vi "spi_control.vi"(0 "connection ID":refnum<k5>, 1 "Device":u16(ring) items=["Attenuation", "Clipping", "Enable channel", "Delay line", "ASIC"], 2 "Read/#write":bool, 3 "Data":i32=72, 4 "Register or channel":i32=72, 5 "error out 3":errorcluster, 6 "Read physical":bool, 7 "Id in":i32, 8 "chip delay":i32) -> (9 "Data to send hex":string, 11 "Data to send dec":u32, 13 "hex integer string":string, 14 "connection ID out":refnum<k5>, 15 "Id out":i32=72, 16 "data out serial":string, 17 "data read value":u32, 19 "error out 2":errorcluster)   [LabVIEW 2009]
panel:
  out "Data out":string
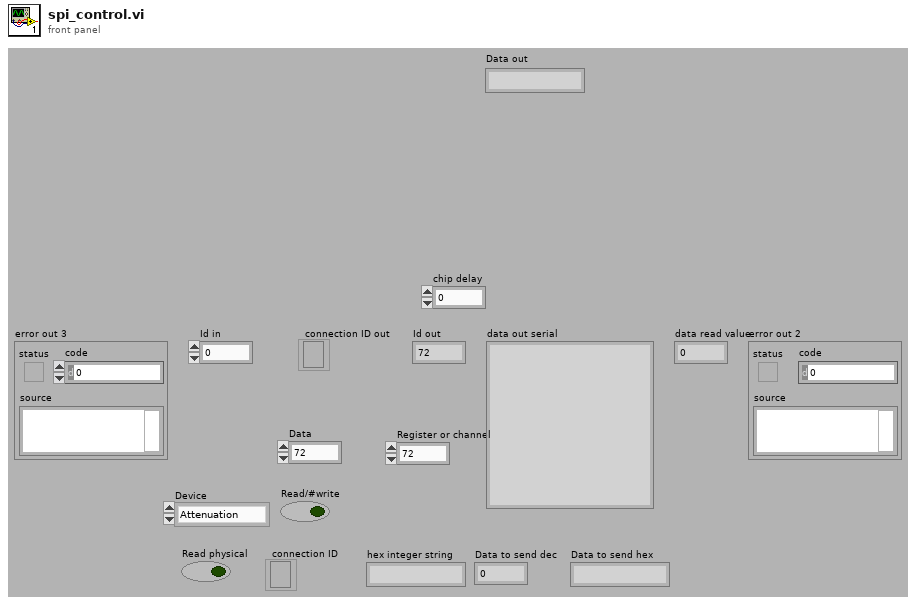
[diagram p1: front panel]
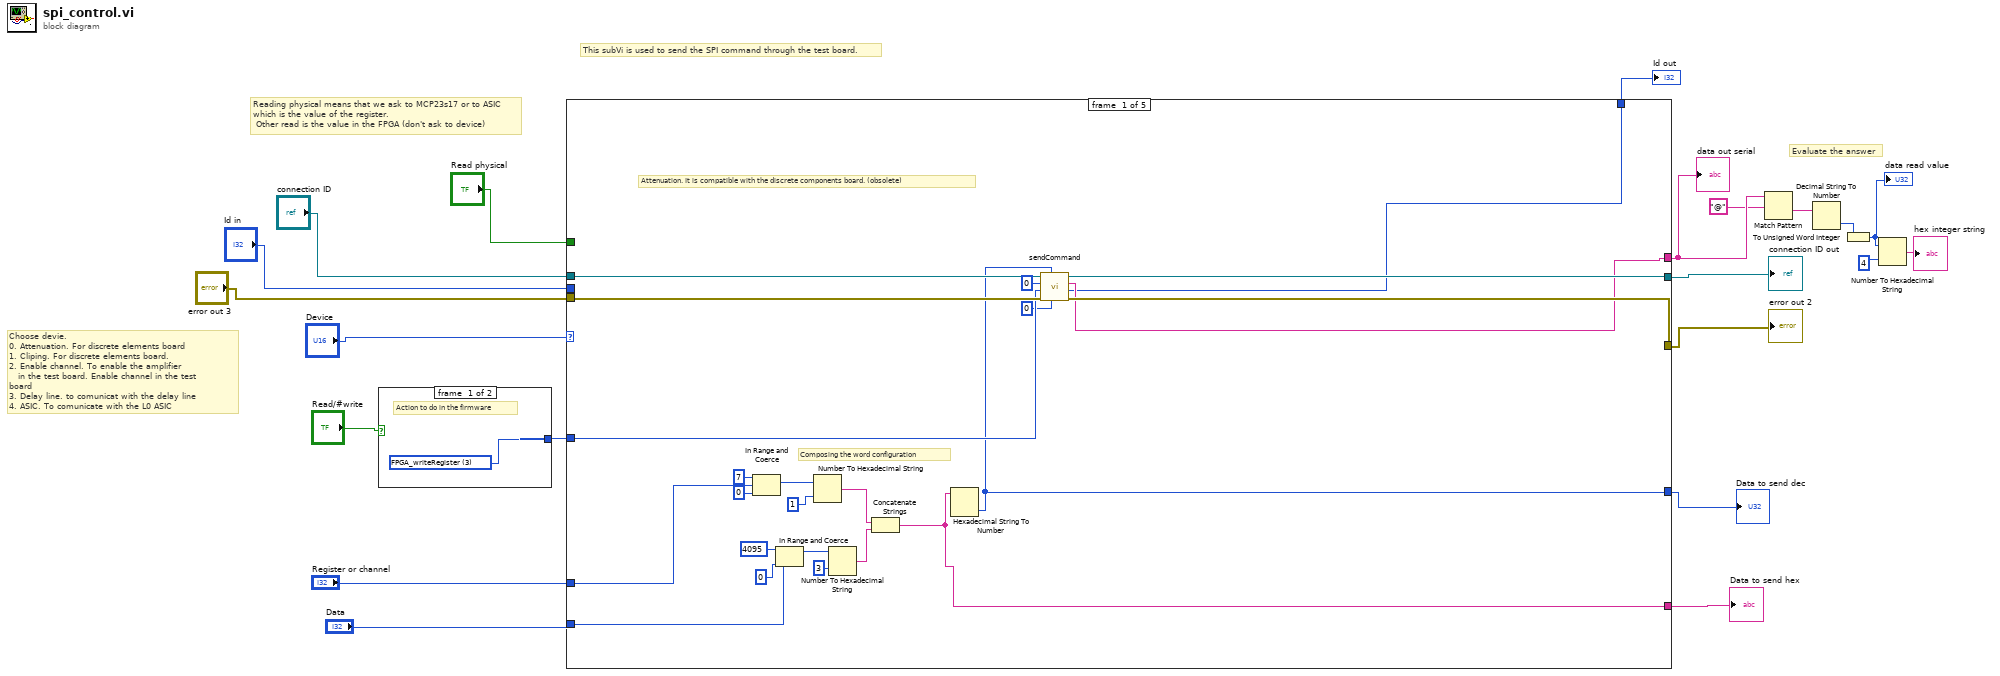
[diagram p0: block diagram]
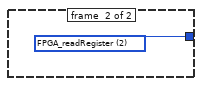
[diagram p2: hidden frame]
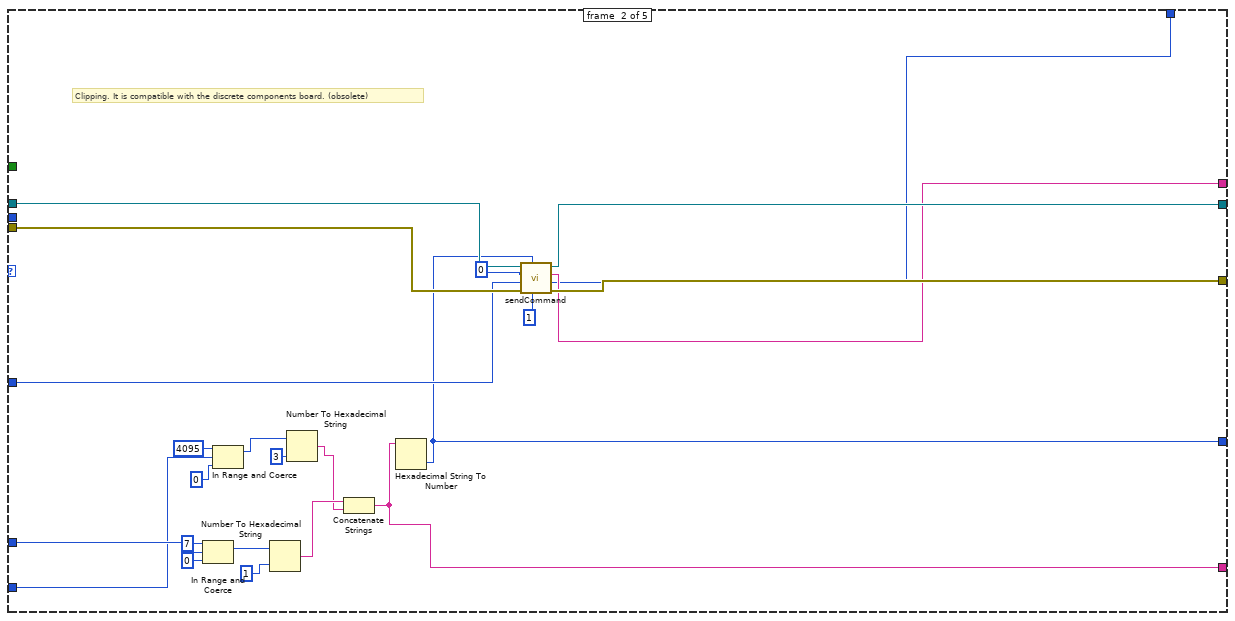
[diagram p3: hidden frame]
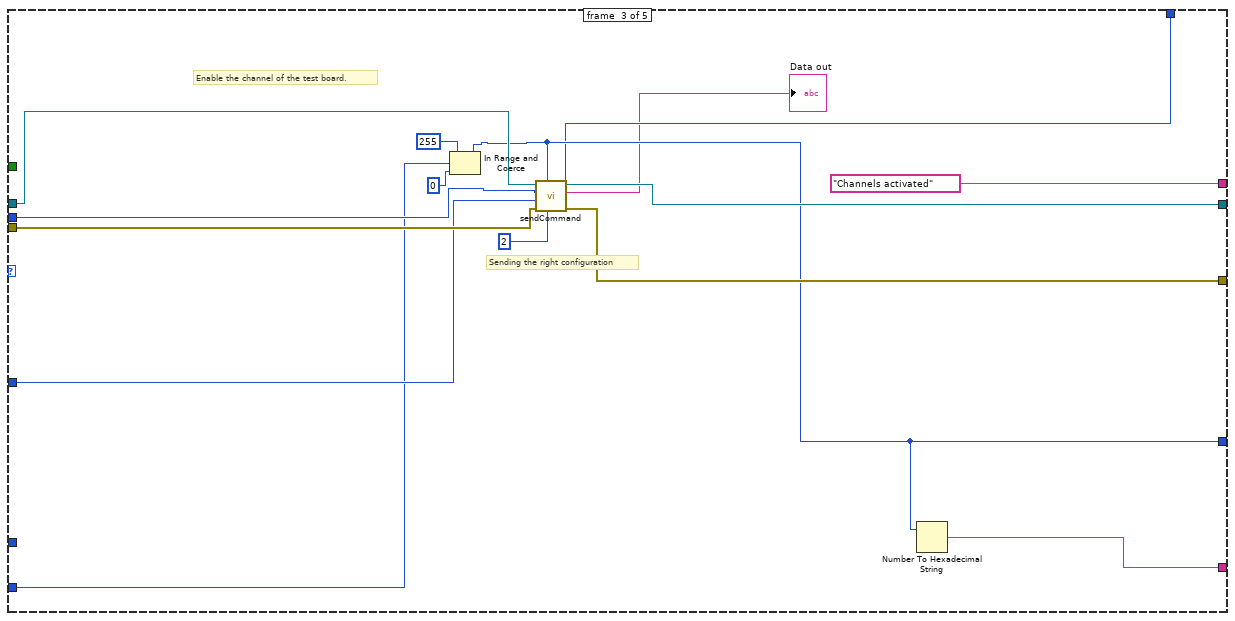
[diagram p4: hidden frame]
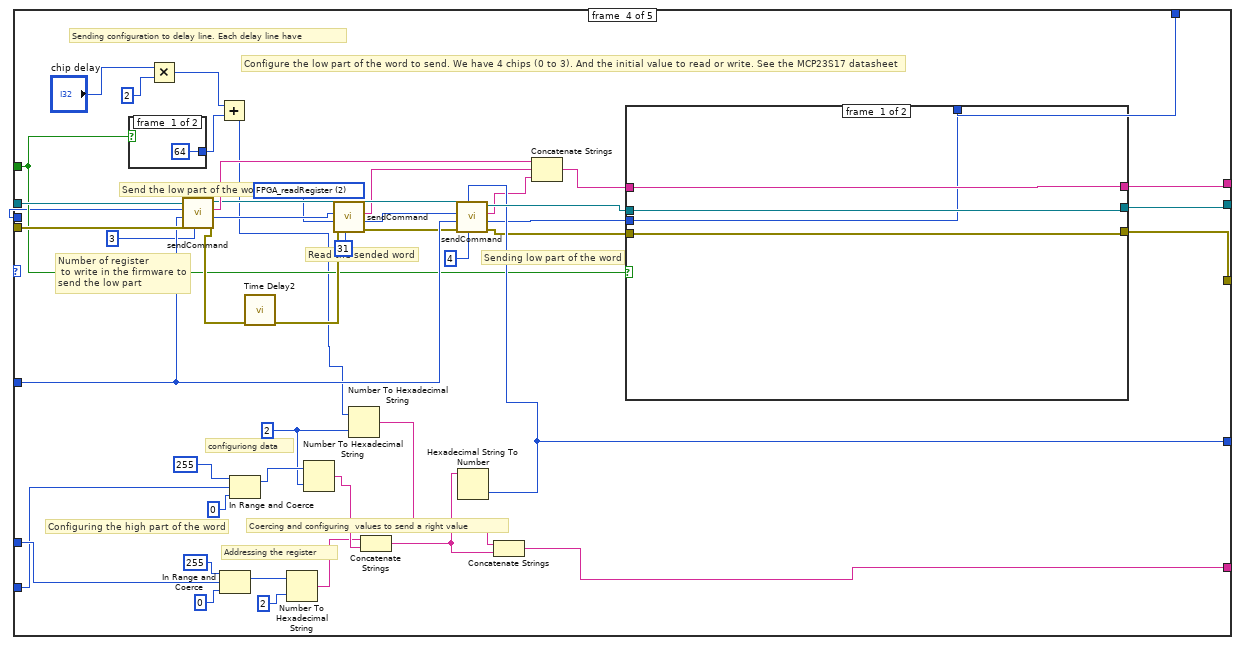
[diagram p5: hidden frame]
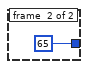
[diagram p6: hidden frame]
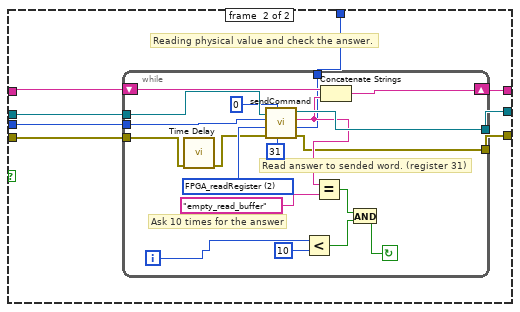
[diagram p7: hidden frame]
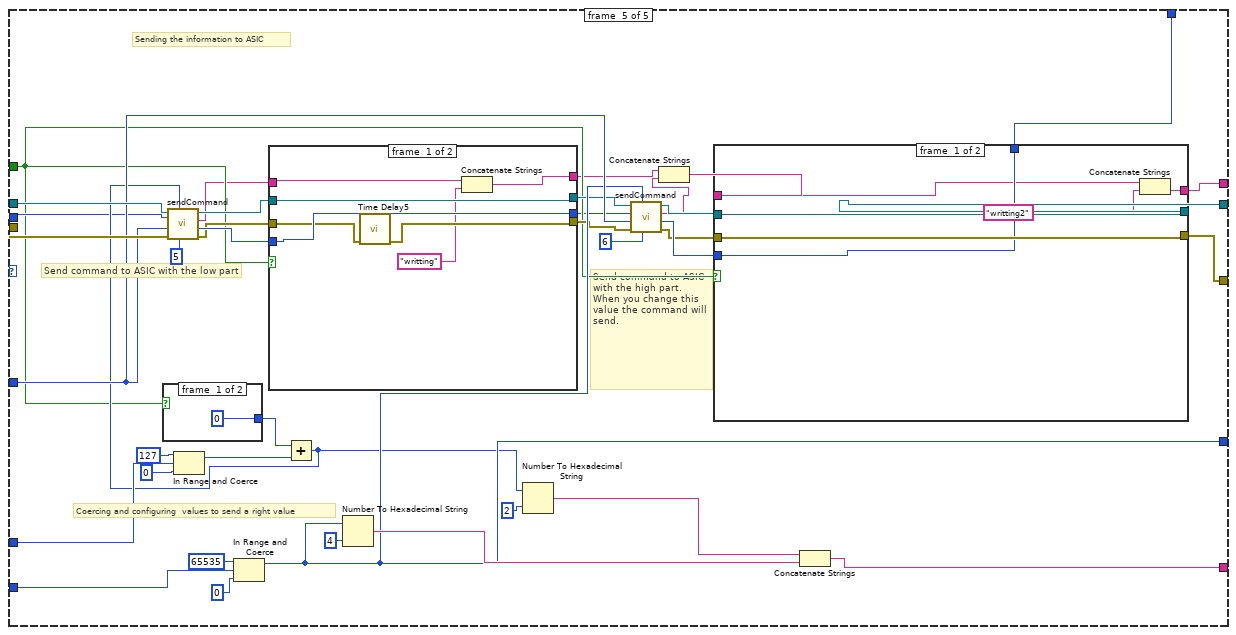
[diagram p8: hidden frame]
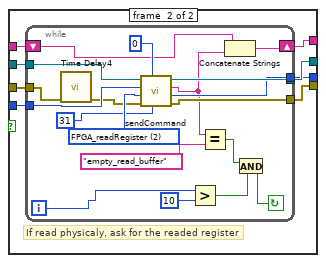
[diagram p9: hidden frame]
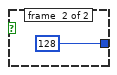
[diagram p10: hidden frame]
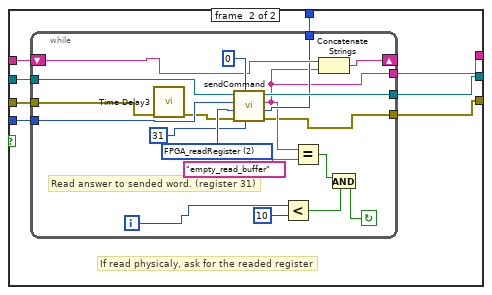
[diagram p11: hidden frame]
diagram:
  # "Reading physical means that we ask to MCP23s17 or to ASIC \nwhich is the value of the register.\n Other read is the value in the FPGA (don't ask to device)"
  # "Evaluate the answer"
  # "Choose devie.\n0. Attenuation. For discrete elements board\n1. Cliping. For discrete elements board.\n2. Enable channel. To enable the amplifier \n   in the test board. Enable channel in the test board\n3. Delay line. to comunicat with the delay line\n4. ASIC. To comunicate with the L0 ASIC"
  # "This subVi is used to send the SPI command through the test board."
  n1 = case shown="False" "Read/#write" {
    tunnel: [w22 w23] -> w9
    frame #0 {
      w22 = u16 3 items=["sendCommand"=9, "FPGA_writeRegister"=3, "FPGA_readRegister"=2, "uC_writeRegister"=1, "uC_readRegister"=0] ("Action")
      # "Action to do in the firmware"
    }
    frame #1 {
      w23 = u16 2 items=["sendCommand"=9, "FPGA_writeRegister"=3, "FPGA_readRegister"=2, "uC_writeRegister"=1, "uC_readRegister"=0] ("Action")
    }
  }
  n2 = case shown="3" "Device" {
    tunnel: [w44 w67 w80 w106 w179] -> w7
    tunnel: "error out 3" -> [w45 w69 w83 w132 w192]
    tunnel: "connection ID" -> [w46 w68 w82 w131 w193]
    tunnel: [w43 w66 w81 w105 w187] -> w6
    tunnel: w9 -> [w31 w63 w79 w130 w191]
    tunnel: "Register or channel" -> [w26 w62 _ w118 w189]
    tunnel: "Data" -> [w27 w57 w75 w117 w190]
    tunnel: [w25 w48 "Channels activated" ("data out") w104 w180] -> w18
    tunnel: [w29 w50 w74 w116 w184] -> w13
    tunnel: [w28 w49 w72 w111 w188] -> w14
    tunnel: "Read physical" -> [_ _ _ w91 w172]
    tunnel: "Id in" -> [_ _ w78 w85 w182]
    tunnel: [w24 w47 w71 w92 w170] -> w3
    frame #0 {
      # "Attenuation. It is compatible with the discrete components board. (obsolete)"
      # "Composing the word configuration"
      n3 = In Range and Coerce(upper limit=7, x=w26, lower limit=0) -> (coerced(x)=w41:i32)  [unwired: 1 out]
      n4 = In Range and Coerce(upper limit=4095, x=w27, lower limit=0) -> (coerced(x)=w37:i32)  [unwired: 1 out]
      n5 = Number To Hexadecimal String(1:i16 1 ("width (-)"), 2:w41) -> (0:w34:string)
      n6 = Number To Hexadecimal String(1:i16 3 ("width (-)"), 2:w37) -> (0:w33:string)
      n7 = Concatenate Strings(w34, w33) -> (w28:string)
      n8 = Hexadecimal String To Number(string=w28) -> (number=w29:u32)  [unwired: 2 in, 1 out]
      n9 = call "sendCommand.vi"("Address"=0, "Data"=w29, "error in"=w45, "Action"=w31, "id_in"=0, "connection ID"=w46) -> ("error out"=w44:errorcluster, "id_out"=w24:i32, "Data out"=w25:string, "connection ID out"=w43:refnum<k5>)  [unwired: 1 in, 1 out]
    }
    frame #1 {
      # "Clipping. It is compatible with the discrete components board. (obsolete)"
      n10 = In Range and Coerce(upper limit=7, x=w62, lower limit=0) -> (coerced(x)=w61:i32)  [unwired: 1 out]
      n11 = In Range and Coerce(upper limit=4095, x=w57, lower limit=0) -> (coerced(x)=w56:i32)  [unwired: 1 out]
      n12 = Number To Hexadecimal String(1:i16 1 ("width (-)"), 2:w61) -> (0:w53:string)
      n13 = Number To Hexadecimal String(1:i16 3 ("width (-)"), 2:w56) -> (0:w52:string)
      n14 = Concatenate Strings(w53, w52) -> (w49:string)
      n15 = Hexadecimal String To Number(string=w49) -> (number=w50:u32)  [unwired: 2 in, 1 out]
      n16 = call "sendCommand.vi"("Address"=1, "Data"=w50, "error in"=w69, "Action"=w63, "id_in"=0 ("id"), "connection ID"=w68) -> ("error out"=w67:errorcluster, "id_out"=w47:i32, "Data out"=w48:string, "connection ID out"=w66:refnum<k5>)  [unwired: 1 in, 1 out]
    }
    frame #2 {
      # "Sending the right configuration"
      # "Enable the channel of the test board."
      n17 = In Range and Coerce(upper limit=255, x=w75, lower limit=0) -> (coerced(x)=w74:i32)  [unwired: 1 out]
      n18 = call "sendCommand.vi"("Address"=2, "Data"=w74, "error in"=w83, "Action"=w79, "id_in"=w78, "connection ID"=w82) -> ("error out"=w80:errorcluster, "id_out"=w71:i32, "Data out"=→"Data out":string, "connection ID out"=w81:refnum<k5>)  [unwired: 1 in, 1 out]
      n19 = Number To Hexadecimal String(2:w74) -> (0:w72:string)  [unwired: 1 in]
    }
    frame #3 {
      w97 = u16 2 items=["sendCommand"=9, "FPGA_writeRegister"=3, "FPGA_readRegister"=2, "uC_writeRegister"=1, "uC_readRegister"=0] ("Action")
      w114 = i16 2 ("width (-)")
      # "Coercing and configuring  values to send a right value"
      # "Number of register\n to write in the firmware to \nsend the low part"
      # "Sending low part of the word"
      # "configuriong data"
      # "Addressing the register"
      # "Configuring the high part of the word"
      # "Read the sended word"
      # "Send the low part of the word"
      # "Configure the low part of the word to send. We have 4 chips (0 to 3). And the initial value to read or write. See the MCP23S17 datasheet"
      # "Sending configuration to delay line. Each delay line have"
      n20 = case shown="False" w91 {
        tunnel: [64 ("Address") 65 ("Address")] -> w88
        frame #0 {
        }
        frame #1 {
        }
      }
      n21 = Multiply(x="chip delay", y=2) -> (x*y=w89:i32)
      n22 = Add(x=w89, y=w88) -> (x+y=w87:i32)
      n23 = call "sendCommand.vi"("Address"=3, "Data"=w87, "error in"=w132, "Action"=w130, "id_in"=w85, "connection ID"=w131) -> ("error out"=w93:errorcluster, "id_out"=w100:i32, "Data out"=w110:string, "connection ID out"=w102:refnum<k5>)  [unwired: 1 in, 1 out]
      n24 = In Range and Coerce(upper limit=255, x=w118, lower limit=0) -> (coerced(x)=w126:i32)  [unwired: 1 out]
      n25 = In Range and Coerce(upper limit=255, x=w117, lower limit=0) -> (coerced(x)=w122:i32)  [unwired: 1 out]
      n26 = call "Time Delay2"("error in (no error)"=w93) -> ("error out"=w94:errorcluster)  [unwired: 10 in]
      n27 = Number To Hexadecimal String(1:i16 2 ("width (-)"), 2:w126) -> (0:w115:string)
      n28 = Number To Hexadecimal String(1:w114, 2:w122) -> (0:w119:string)
      n29 = call "sendCommand.vi"("Address"=31, "error in"=w94, "Action"=w97, "id_in"=w100, "connection ID"=w102) -> ("error out"=w103:errorcluster, "id_out"=w99:i32, "Data out"=w98:string, "connection ID out"=w101:refnum<k5>)  [unwired: 2 in, 1 out]
      n30 = Number To Hexadecimal String(1:w114, 2:w87) -> (0:w113:string)
      n31 = Concatenate Strings(w115, w119) -> (w112:string)
      n32 = Hexadecimal String To Number(string=w112) -> (number=w116:u32)  [unwired: 2 in, 1 out]
      n33 = call "sendCommand.vi"("Address"=4, "Data"=w116, "error in"=w103, "Action"=w130, "id_in"=w99, "connection ID"=w101) -> ("error out"=w95:errorcluster, "id_out"=w107:i32, "Data out"=w109:string, "connection ID out"=w127:refnum<k5>)  [unwired: 1 in, 1 out]
      n34 = Concatenate Strings(w113, w112) -> (w111:string)
      n35 = Concatenate Strings(w110, w98, w109) -> (w108:string)
      n36 = case shown="False" w91 {
        tunnel: w127 -> [w137 w146]
        tunnel: w95 -> [w138 w145]
        tunnel: [w138 w142] -> w106
        tunnel: [w137 w143] -> w105
        tunnel: [w136 w144] -> w104
        tunnel: w108 -> [w136 w141]
        tunnel: w107 -> [w135 w140]
        tunnel: [w135 w139] -> w92
        frame #0 {
        }
        frame #1 {
          # "Reading physical value and check the answer."
          n37 = while {
            tunnel: w145 -> [w149]
            tunnel: [w150] -> w142
            tunnel: [w155] -> w143
            tunnel: w146 -> [w159]
            shift-right: [w152] -> w144
            shift-left: w141 -> [w154]
            tunnel: w140 -> [w151]
            tunnel: [w147] -> w139
            i -> [w160]
            stop <- w161 continue-if-true
            w158 = u16 2 items=["sendCommand"=9, "FPGA_writeRegister"=3, "FPGA_readRegister"=2, "uC_writeRegister"=1, "uC_readRegister"=0] ("Action 2")
            # "Read answer to sended word. (register 31)"
            # "Ask 10 times for the answer"
            n38 = call "Time Delay"("error in (no error)"=w149) -> ("error out"=w148:errorcluster)  [unwired: 10 in]
            n39 = call "sendCommand.vi"("Address"=31, "Data"=0, "error in"=w148, "Action"=w158, "id_in"=w151, "connection ID"=w159) -> ("error out"=w150:errorcluster, "id_out"=w147:i32, "Data out"=w153:string, "connection ID out"=w155:refnum<k5>)  [unwired: 1 in, 1 out]
            n40 = Less?(x=w160, y=10) -> (x < y?=w163:bool)
            n41 = Equal?(x=w153, y="empty_read_buffer") -> (x = y?=w164:bool)
            n42 = Concatenate Strings(w154, w153) -> (w152:string)
            n43 = And(x=w164, y=w163) -> (x .and. y?=w161:bool)
          }
        }
      }
    }
    frame #4 {
      # "Coercing and configuring  values to send a right value"
      # "Send command to ASIC with the high part. When you change this value the command will send."
      # "Send command to ASIC with the low part"
      # "Sending the information to ASIC"
      n44 = case shown="True" w172 {
        tunnel: [0 ("Address") 128 ("Address")] -> w186
        frame #0 {
        }
        frame #1 {
        }
      }
      n45 = In Range and Coerce(upper limit=127, x=w189, lower limit=0) -> (coerced(x)=w185:i32)  [unwired: 1 out]
      n46 = In Range and Coerce(upper limit=65535, x=w190, lower limit=0) -> (coerced(x)=w184:i32)  [unwired: 1 out]
      n47 = Add(x=w186, y=w185) -> (x+y=w183:i32)
      n48 = call "sendCommand.vi"("Address"=5, "Data"=w183, "error in"=w192, "Action"=w191, "id_in"=w182, "connection ID"=w193) -> ("error out"=w173:errorcluster, "id_out"=w175:i32, "Data out"=w166:string, "connection ID out"=w174:refnum<k5>)  [unwired: 1 in, 1 out]
      n49 = case shown="True" w172 {
        tunnel: w174 -> [w211 w219]
        tunnel: w173 -> [w209 w218]
        tunnel: [w208 w217] -> w177
        tunnel: [w211 w216] -> w176
        tunnel: [w206 w214] -> w169
        tunnel: w175 -> [w210 w215]
        tunnel: [w210 w213] -> w171
        tunnel: w166 -> [w205 w212]
        frame #0 {
          n50 = call "Time Delay5"("error in (no error)"=w209) -> ("error out"=w208:errorcluster)  [unwired: 10 in]
          n51 = Concatenate Strings(w205, "writting" ("Data out")) -> (w206:string)
        }
        frame #1 {
          # "If read physicaly, ask for the readed register"
          n52 = while {
            tunnel: w218 -> [w226]
            tunnel: [w224] -> w217
            tunnel: [w232] -> w216
            tunnel: w219 -> [w228]
            tunnel: w215 -> [w231]
            tunnel: [w223] -> w213
            shift-right: [w220] -> w214
            shift-left: w212 -> [w222]
            i -> [w233]
            stop <- w234 continue-if-true
            w230 = u16 2 items=["sendCommand"=9, "FPGA_writeRegister"=3, "FPGA_readRegister"=2, "uC_writeRegister"=1, "uC_readRegister"=0] ("Action 2")
            n53 = call "Time Delay4"("error in (no error)"=w226) -> ("error out"=w225:errorcluster)  [unwired: 10 in]
            n54 = call "sendCommand.vi"("Address"=31, "Data"=0, "error in"=w225, "Action"=w230, "id_in"=w231, "connection ID"=w228) -> ("error out"=w224:errorcluster, "id_out"=w223:i32, "Data out"=w221:string, "connection ID out"=w232:refnum<k5>)  [unwired: 1 in, 1 out]
            n55 = Greater?(x=w233, y=10) -> (0:w236:bool)
            n56 = Equal?(x=w221, y="empty_read_buffer") -> (x = y?=w237:bool)
            n57 = Concatenate Strings(w222, w221) -> (w220:string)
            n58 = And(x=w237, y=w236) -> (x .and. y?=w234:bool)
          }
        }
      }
      n59 = Number To Hexadecimal String(1:i16 4 ("width (-)"), 2:w184) -> (0:w194:string)
      n60 = Number To Hexadecimal String(1:i16 2 ("width (-)"), 2:w183) -> (0:w195:string)
      n61 = call "sendCommand.vi"("Address"=6, "Data"=w184, "error in"=w177, "Action"=w191, "id_in"=w171, "connection ID"=w176) -> ("error out"=w178:errorcluster, "id_out"=w181:i32, "Data out"=w168:string, "connection ID out"=w202:refnum<k5>)  [unwired: 1 in, 1 out]
      n62 = Concatenate Strings(w169, w168) -> (w167:string)
      n63 = case shown="True" w172 {
        tunnel: w202 -> [w245 w254]
        tunnel: w178 -> [w246 w253]
        tunnel: [w246 w252] -> w179
        tunnel: [w245 w251] -> w187
        tunnel: [w243 w247] -> w180
        tunnel: w181 -> [w244 w250]
        tunnel: w167 -> [w241 w249]
        tunnel: [w244 w248] -> w170
        frame #0 {
          n64 = Concatenate Strings(w241, "writting2" ("Data out")) -> (w243:string)
        }
        frame #1 {
          # "If read physicaly, ask for the readed register"
          n65 = while {
            tunnel: w253 -> [w261]
            tunnel: [w255] -> w252
            tunnel: [w267] -> w251
            tunnel: w254 -> [w263]
            tunnel: w250 -> [w266]
            tunnel: [w257] -> w248
            shift-right: [w259] -> _
            shift-left: w249 -> [w258]
            tunnel: [w256] -> w247
            i -> [w268]
            stop <- w269 continue-if-true
            w265 = u16 2 items=["sendCommand"=9, "FPGA_writeRegister"=3, "FPGA_readRegister"=2, "uC_writeRegister"=1, "uC_readRegister"=0] ("Action 2")
            # "Read answer to sended word. (register 31)"
            n66 = call "Time Delay3"("error in (no error)"=w261) -> ("error out"=w260:errorcluster)  [unwired: 10 in]
            n67 = call "sendCommand.vi"("Address"=31, "Data"=0, "error in"=w260, "Action"=w265, "id_in"=w266, "connection ID"=w263) -> ("error out"=w255:errorcluster, "id_out"=w257:i32, "Data out"=w256:string, "connection ID out"=w267:refnum<k5>)  [unwired: 1 in, 1 out]
            n68 = Less?(x=w268, y=10) -> (x < y?=w271:bool)
            n69 = Equal?(x=w256, y="empty_read_buffer") -> (x = y?=w272:bool)
            n70 = Concatenate Strings(w258, w256) -> (w259:string)
            n71 = And(x=w272, y=w271) -> (x .and. y?=w269:bool)
          }
        }
      }
      n72 = Concatenate Strings(w195, w194) -> (w188:string)
    }
  }
  "data out serial" <- w18
  "Data to send dec" <- w13
  "Data to send hex" <- w14
  "Id out" <- w3
  "error out 2" <- w7
  "connection ID out" <- w6
  n73 = Match Pattern(string=w18, regular expression="@" ("search string/char (-)")) -> (after substring=w16:string)  [unwired: 1 in, 3 out]
  n74 = Decimal String To Number(string=w16) -> (number=w2:i32)  [unwired: 2 in, 1 out]
  n75 = To Unsigned Word Integer(number=w2) -> (unsigned 16bit integer=w1:u16)
  "data read value" <- w1
  n76 = Number To Hexadecimal String(1:i16 4 ("width (-)"), 2:w1) -> (0:→"hex integer string":string)
